vi "Stats Unbundle v0.2.vi"(8 "NAT Cluster in":T2, 9 "State":T4, 10 "Model":string, 11 "Auto Stats":T6) -> (0 "NAT Cluster out":T1, 1 "Cycle Time":dbl, 2 "Counters":cluster{"GoodCount":u32, "RejectCount":u32}, 3 "OEE Cluster":T3, 4 "Avg. Cycle Time":dbl, 5 "Total Times":T5, 7 "path":path)   [LabVIEW 2021]
doc: "v0.2:\n- Added state for saving and loading values"
uses:
  support/Controls/Auto Stats.ctl
  RT/Controls/Auto Times.ctl
  Controls/Logging FGV.ctl
  Controls/AVL Auto Time.ctl
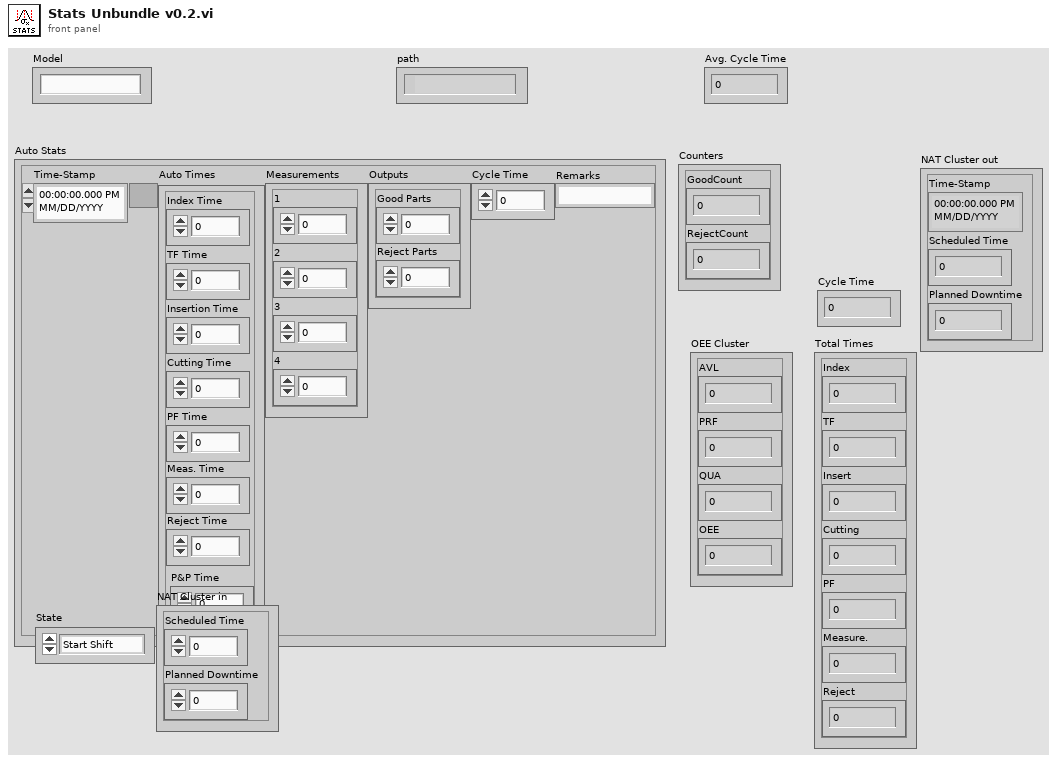
[diagram p1: front panel]
types:
  T1 = cluster{"Time-Stamp":timestamp, "Scheduled Time":dbl, "Planned Downtime":dbl}
  T2 = cluster{"Scheduled Time":dbl, "Planned Downtime":dbl}
  T3 = cluster{"AVL":dbl, "PRF":dbl, "QUA":dbl, "OEE":dbl}
  T4 = typedef "Logging FGV.ctl" = enum16{"Start Shift", "Reload Values", "Log Index", "Read Shift", "Close Shift", "Save Values"}
  T5 = cluster{"Index":dbl, "TF":dbl, "Insert":dbl, "Cutting":dbl, "PF":dbl, "Measure.":dbl, "Reject":dbl}
  T6 = typedef "Auto Stats.ctl" = cluster{"Time-Stamp":timestamp, "Auto Times":T7, "Measurements":cluster{"1":dbl, "2":dbl, "3":dbl, "4":dbl}, "Outputs":cluster{"Good Parts":u32, "Reject Parts":u32}, "Cycle Time":dbl, "Remarks":string}
  T7 = typedef "Auto Times.ctl" = cluster{"Index Time":u32, "TF Time":u32, "Insertion Time":u32, "Cutting Time":u32, "PF Time":u32, "Meas. Time":u32, "Reject Time":u32, "P&P Time":u32}
  T8 = typedef "AVL Auto Time.ctl" = enum16{"Start Session", "Exited Auto", "Resumed Auto", "Read Time", "Reload Values"}
  T9 = cluster{"[0]":dbl, "[1]":dbl, "[2]":dbl, "[3]":dbl, "[4]":dbl, "[5]":dbl, "[6]":dbl}
  T10 = cluster{"value":dbl, "value":dbl, "value":dbl, "value":dbl}
  T11 = cluster{"Time of Exit":timestamp, "value":dbl, "value":dbl}
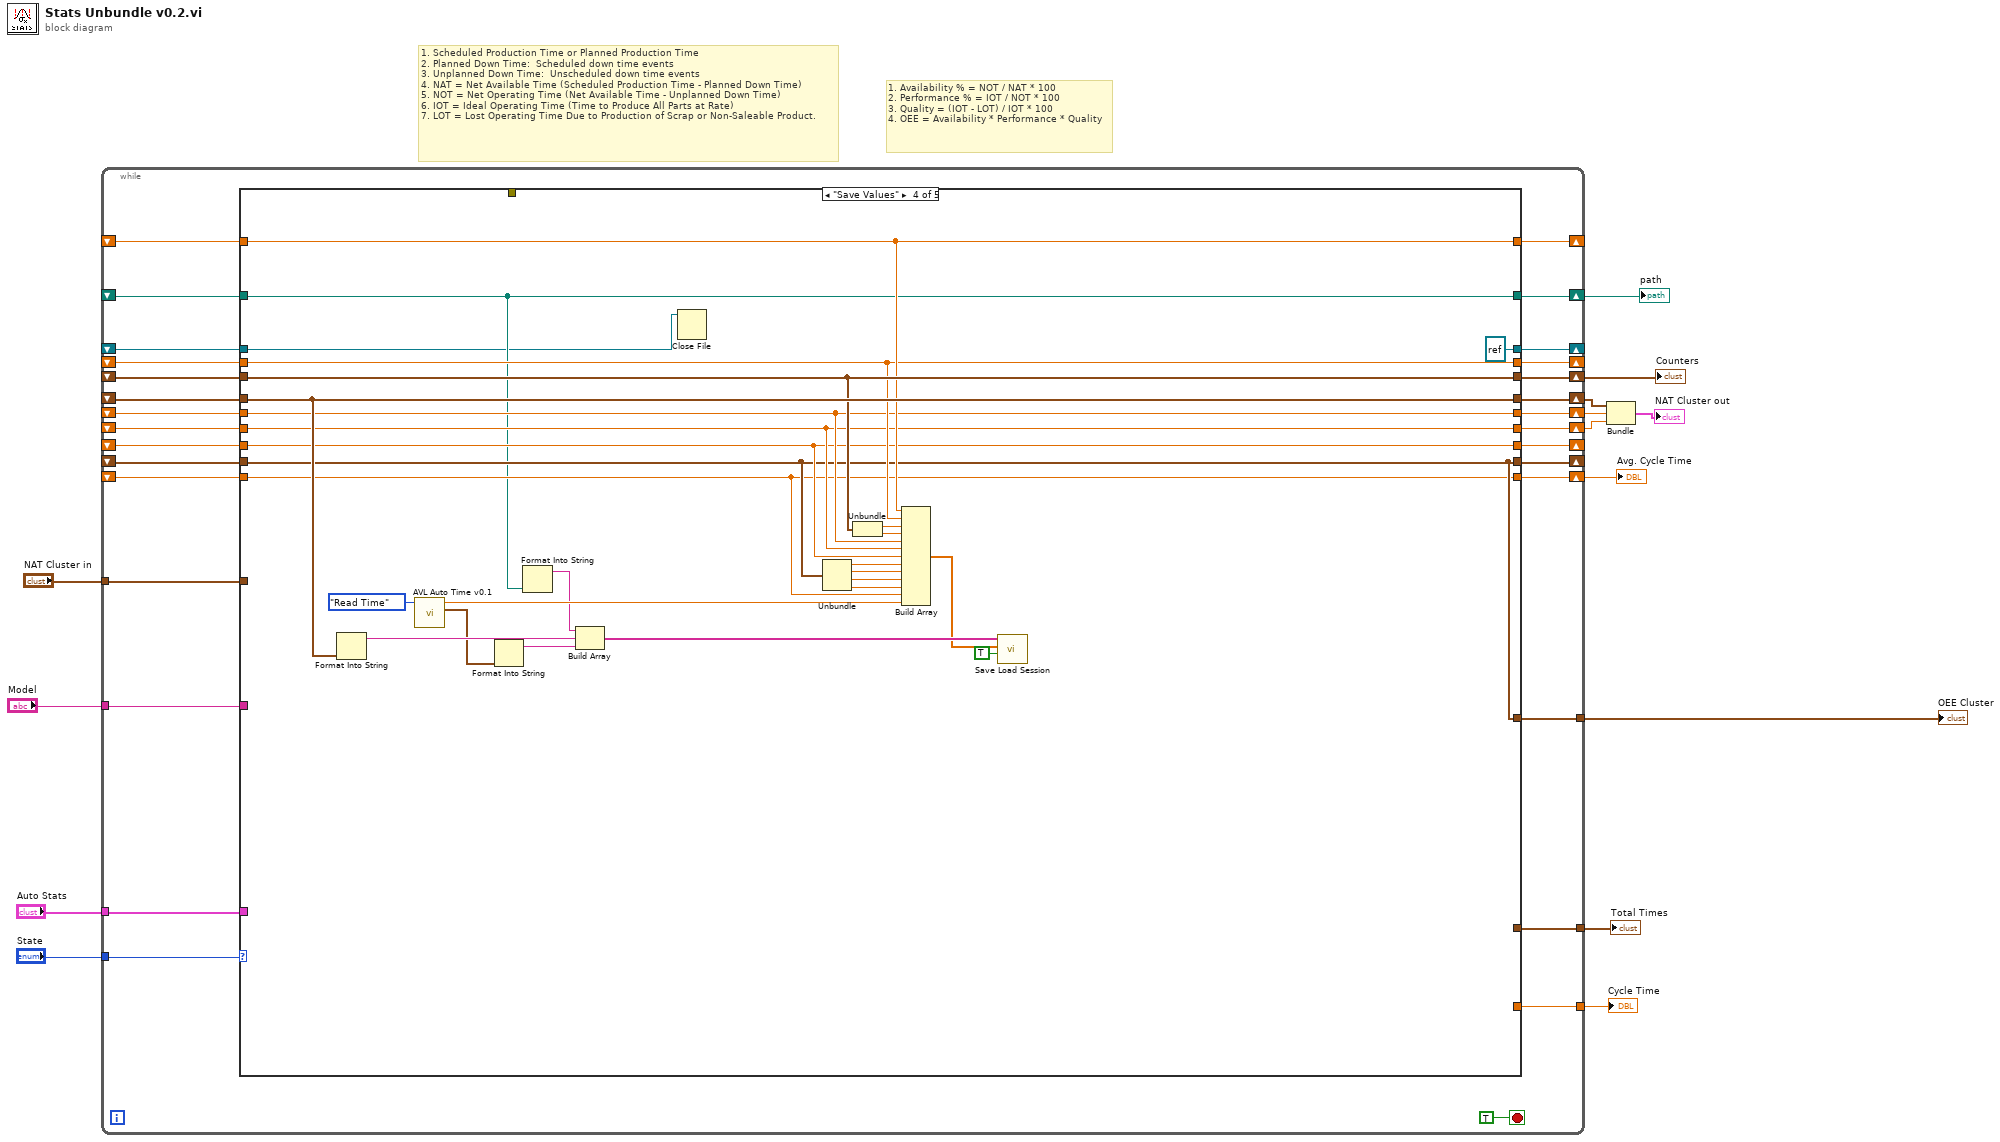
[diagram p0: block diagram]
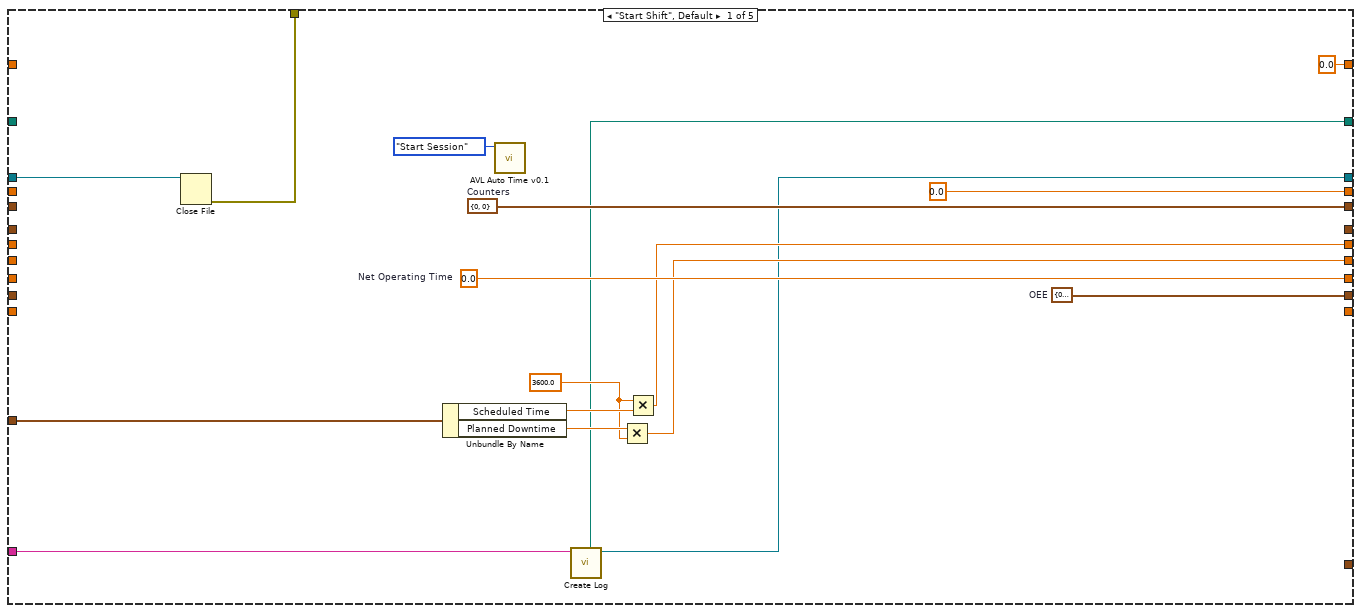
[diagram p2: hidden frame]
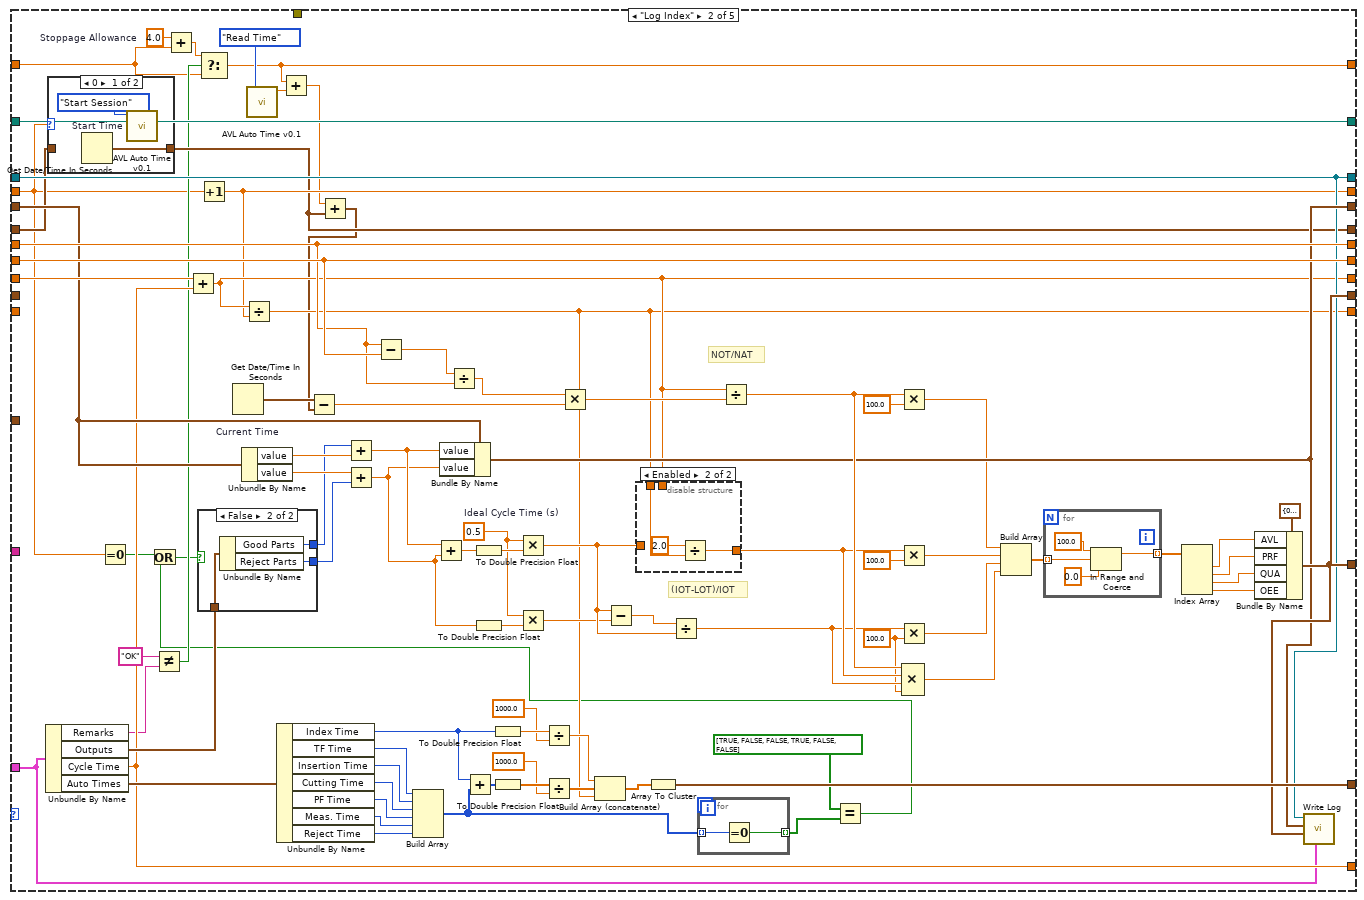
[diagram p3: hidden frame]
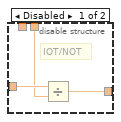
[diagram p4: hidden frame]
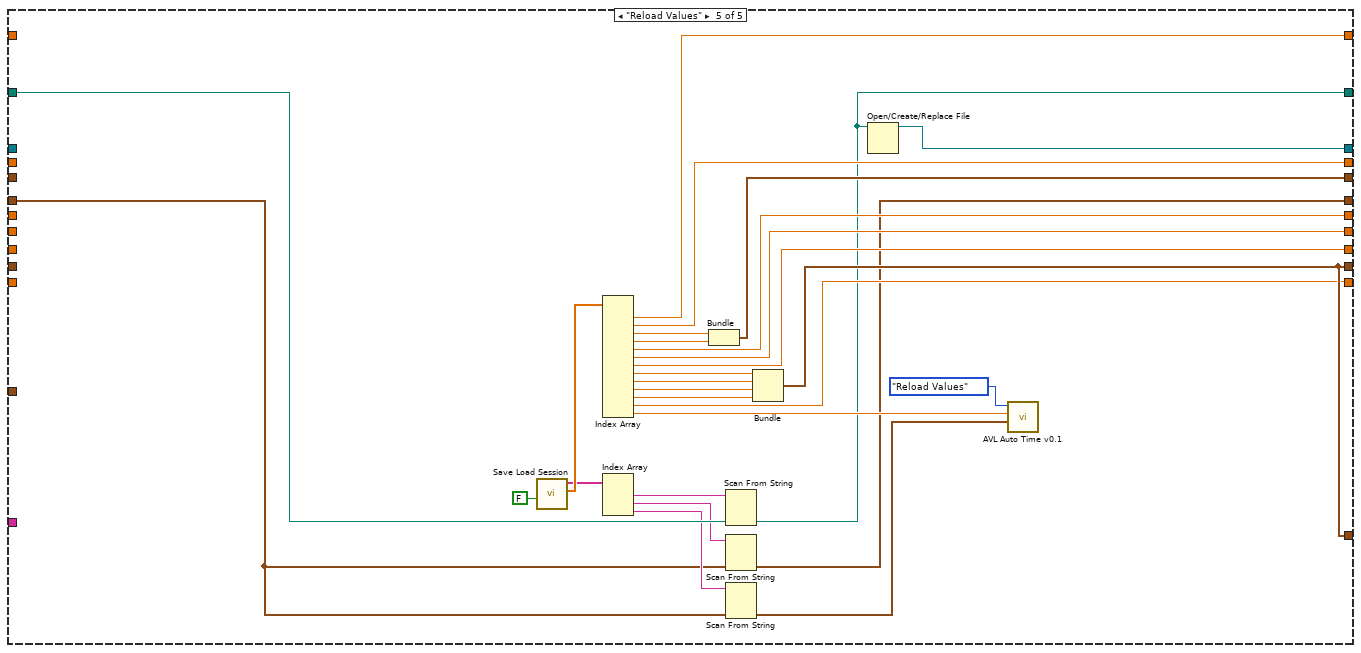
[diagram p8: hidden frame]
diagram:
  # "1.\tAvailability % = NOT / NAT * 100\n2.\tPerformance % = IOT / NOT * 100\n3.\tQuality = (IOT - LOT) / IOT * 100\n4.\tOEE = Availability * Performance * Quality"
  # "1.\tScheduled Production Time or Planned Production Time\n2.\tPlanned Down Time:  Scheduled down time events\n3.\tUnplanned Down Time:  Unscheduled down time events\n4.\tNAT = Net Available Time (Scheduled Production Time - Planned Down Time)\n5.\tNOT = Net Operating Time (Net Available Time - Unplanned Down Time)\n6.\tIOT = Ideal Operating Time (Time to Produce All Parts at Rate)\n7.\tLOT = Lost Operating Time Due to Production of Scrap or Non-Saleable Product."
  n1 = while {
    tunnel: "Auto Stats" -> [w44]
    tunnel: "State" -> [w43]
    shift-right: [w40] -> w8
    shift-left: _ -> [w37]
    shift-right: [w41] -> w9
    shift-left: _ -> [w38]
    shift-right: [w42] -> w6
    shift-left: _ -> [w39]
    shift-right: [w36] -> _
    shift-left: _ -> [w35]
    tunnel: [w34] -> w2
    shift-right: [w33] -> w13
    shift-left: _ -> [w32]
    tunnel: [w31] -> w12
    tunnel: [w29] -> w11
    shift-right: [w28] -> _
    shift-left: _ -> [w27]
    tunnel: "NAT Cluster in" -> [w26]
    shift-right: [w25] -> _
    shift-left: _ -> [w24]
    tunnel: "Model" -> [w23]
    shift-right: [w22] -> _
    shift-left: _ -> [w21]
    shift-right: [w20] -> w3
    shift-left: _ -> [w19]
    shift-right: [w18] -> w1
    shift-left: _ -> [w17]
    shift-right: [w16] -> _
    shift-left: _ -> [w15]
    stop <- TRUE stop-if-true
    n2 = case shown="\"Save Values\"" w43 {
      tunnel: w44 -> [_ w100 _ _ _]
      tunnel: [_ w79 w176 w202 w207] -> w42
      tunnel: [w54 w115 w173 w196 w222] -> w41
      tunnel: [w55 w130 w175 w195 w223] -> w40
      tunnel: w39 -> [_ w94 w176 w202 w204]
      tunnel: w38 -> [_ w115 w173 w196 _]
      tunnel: w37 -> [_ w130 w175 w195 _]
      tunnel: [w61 w96 w174 w194 w224] -> w36
      tunnel: w35 -> [_ w125 w174 w194 _]
      tunnel: [_ w99 w171 w193 w217] -> w34
      tunnel: [w60 w98 w172 w201 w225] -> w33
      tunnel: w32 -> [_ w105 w172 w201 _]
      tunnel: [_ w102 _ _ _] -> w31
      tunnel: [_ w101 _ _ _] -> w29
      tunnel: [w59 w99 w171 w193 w217] -> w28
      tunnel: w27 -> [_ _ w171 w193 _]
      tunnel: w26 -> [w56 _ _ _ _]
      tunnel: [w52 w97 w170 refnum<file> refnum ("refnum out") w209] -> w25
      tunnel: w24 -> [w51 w97 w170 w178 _]
      tunnel: [w50 _ _ _ _] -> _
      tunnel: w23 -> [w49 _ _ _ _]
      tunnel: [0.0 w95 w169 w199 w228] -> w22
      tunnel: w21 -> [_ w65 w169 w199 _]
      tunnel: [_ w80 w168 w188 w216] -> w20
      tunnel: w19 -> [_ _ w168 w188 _]
      tunnel: [w47 w83 w167 w186 w210] -> w18
      tunnel: w17 -> [_ w83 w167 w186 w211]
      tunnel: [0.0 w70 w166 w200 w229] -> w16
      tunnel: w15 -> [_ w72 w166 w200 _]
      frame "Start Shift", Default {
        w53 = 3600.0 ("y")
        w59 = T3 {"AVL"=0.0, "PRF"=0.0, "QUA"=0.0, "OEE"=0.0}  # OEE
        w60 = cluster{"GoodCount":u32, "RejectCount":u32} {"GoodCount"=0, "RejectCount"=0}  # Counters
        w61 = 0.0  # Net Operating Time
        n3 = Close File(refnum=w51) -> (error out=w50:errorcluster)  [unwired: 1 in, 1 out]
        n4 = Unbundle By Name(w56) -> ("Scheduled Time"=w58:dbl, "Planned Downtime"=w57:dbl)
        n5 = call "AVL Auto Time v0.1.vi"("State"=AVL_Auto_Time."Start Session") -> ()  [unwired: 9 in, 2 out]
        n6 = call "Create Log.vi"("Model"=w49) -> ("refnum out"=w52:refnum<file>, "path"=w47:path)  [unwired: 9 in]
        n7 = Multiply(x=w57, y=w53) -> (x*y=w55:dbl)
        n8 = Multiply(x=w53, y=w58) -> (x*y=w54:dbl)
      }
      frame "Log Index" {
        w75 = 4.0  # Stoppage Allowance
        w111 = 100.0 ("y")
        w116 = 0.5  # Ideal Cycle Time (s)
        # "NOT/NAT"
        # "(IOT-LOT)/IOT"
        n9 = Unbundle By Name(w100) -> ("Remarks"=w77:string, "Outputs"=w124:cluster{"Good Parts":u32, "Reject Parts":u32}, "Cycle Time"=w102:dbl, "Auto Times"=w147:T7)
        n10 = case shown="0" w65 {
          tunnel: w94 -> [_ w165]
          tunnel: [w164 w165] -> w79
          frame 0 {
            n11 = Get Date/Time In Seconds "Start Time"() -> (seconds since 1Jan1904=w164:timestamp)
            n12 = call "AVL Auto Time v0.1.vi"("State"=AVL_Auto_Time."Start Session") -> ()  [unwired: 9 in, 2 out]
          }
          frame Default {
          }
        }
        n13 = Equal To 0?(x=w65) -> (x = 0?=w64:bool)
        n14 = Not Equal?(x="OK", y=w77) -> (x != y?=w74:bool)
        n15 = Add(x=w75, y=w72) -> (x+y=w73:dbl)
        n16 = Add(x=w125, y=w102) -> (x+y=w96:dbl)
        n17 = Select(t=w73, s=w74, f=w72) -> (s? t:f=w70:dbl)
        n18 = Increment(x=w65) -> (x+1=w95:dbl)
        n19 = Get Date/Time In Seconds "Current Time"() -> (seconds since 1Jan1904=w131:timestamp)
        n20 = Unbundle By Name(w105) -> ("value"=w109:dbl, "value"=w108:dbl)
        n21 = Divide(x=w96, y=w95) -> (x/y=w80:dbl)
        n22 = call "AVL Auto Time v0.1.vi"("State"=AVL_Auto_Time."Read Time") -> ("Non-Auto Time"=w71:dbl)  [unwired: 9 in, 1 out]
        n23 = Unbundle By Name(w147) -> ("Index Time"=w133:u32, "TF Time"=w141:u32, "Insertion Time"=w142:u32, "Cutting Time"=w143:u32, "PF Time"=w144:u32, "Meas. Time"=w145:u32, "Reject Time"=w146:u32)
        n24 = Add(x=w70, y=w71) -> (x+y=w69:dbl)
        n25 = Add(x=w69, y=w79) -> (x+y=w78:timestamp)
        n26 = Subtract(x=w131, y=w78) -> (x-y=w129:dbl)
        n27 = Subtract(x=w115, y=w130) -> (x-y=w128:dbl)
        n28 = Build Array(w141, w142, w143, w144, w145, w146) -> (w68:u32[])
        n29 = Divide(x=w128, y=w115) -> (x/y=w82:dbl)
        n30 = Add(x=w133, y=w68) -> (x+y=w138:u32[])
        n31 = To Double Precision Float(number=w133) -> (double precision float=w135:dbl)
        n32 = To Double Precision Float(number=w138) -> (double precision float=w140:dbl[])
        n33 = Divide(x=w135, y=1000.0) -> (x/y=w132:dbl)
        n34 = Divide(x=w140, y=1000.0) -> (x/y=w137:dbl[])
        n35 = Multiply(x=w82, y=w129) -> (x*y=w126:dbl)
        n36 = Build Array (concatenate)(w132, w137, w80) -> (w136:dbl[])
        n37 = Array To Cluster(array=w136) -> (cluster=w101:T9)
        n38 = for {
          tunnel: w68 -> [w149] mode=indexing
          tunnel: [w148] -> w67 mode=indexing
          n39 = Equal To 0?(x=w149) -> (x = 0?=w148:bool)
        }
        n40 = Divide(x=w96, y=w126) -> (x/y=w114:dbl)
        n41 = Equal?(x=bool[] [TRUE, FALSE, FALSE, TRUE, FALSE, FALSE], y=w67) -> (x = y?=w63:bool)
        n42 = Or(x=w64, y=w63) -> (x .or. y?=w62:bool)
        n43 = case shown="False" w62 {
          tunnel: w124 -> [_ w160]
          tunnel: [_ w162] -> w107
          tunnel: [_ w161] -> w106
          frame True {
          }
          frame False {
            n44 = Unbundle By Name(w160) -> ("Good Parts"=w162:u32, "Reject Parts"=w161:u32)
          }
        }
        n45 = Add(x=w107, y=w109) -> (x+y=w104:dbl)
        n46 = Add(x=w108, y=w106) -> (x+y=w103:dbl)
        n47 = Add(x=w104, y=w103) -> (x+y=w123:dbl)
        n48 = Bundle By Name(cluster=w105, "value"=w104, "value"=w103) -> (w98:cluster{"value":dbl, "value":dbl})
        n49 = To Double Precision Float(number=w123) -> (double precision float=w122:dbl)
        n50 = To Double Precision Float(number=w103) -> (double precision float=w120:dbl)
        n51 = Multiply(x=w116, y=w122) -> (x*y=w118:dbl)
        n52 = Multiply(x=w116, y=w120) -> (x*y=w117:dbl)
        n53 = Subtract(x=w118, y=w117) -> (x-y=w119:dbl)
        n54 = disable-structure shown="Enabled" {
          disable-tunnel: w118 -> [w152 _]
          disable-tunnel: [w151 w153] -> w113
          disable-tunnel: w96 -> [w150 _]
          disable-tunnel: w80 -> [_ w155]
          frame Disabled {
            # "IOT/NOT"
            n55 = Divide(x=w152, y=w150) -> (x/y=w151:dbl)
          }
          frame Enabled {
            n56 = Divide(x=2.0 ("y"), y=w155) -> (x/y=w153:dbl)
          }
        }
        n57 = Divide(x=w119, y=w118) -> (x/y=w112:dbl)
        n58 = Multiply(x=w114, y=100.0) -> (x*y=w93:dbl)
        n59 = Multiply(x=w113, y=100.0) -> (x*y=w92:dbl)
        n60 = Multiply(x=w112, y=w111) -> (x*y=w91:dbl)
        n61 = Compound Arithmetic op=MULTIPLY(w114, w113, w112, w111) -> (w90:dbl)
        n62 = Build Array(w93, w92, w91, w90) -> (w89:dbl[])
        n63 = for {
          tunnel: w89 -> [w157] mode=indexing
          tunnel: [w156] -> w88 mode=indexing
          n64 = In Range and Coerce(upper limit=100.0, x=w157, lower limit=0.0) -> (coerced(x)=w156:dbl)  [unwired: 1 out]
        }
        n65 = Index Array(array=w88) -> (element #1=w87:dbl, element #2=w86:dbl, element #3=w85:dbl, element #4=w84:dbl)  [unwired: 4 in]
        n66 = Bundle By Name(cluster=T3 {"AVL"=0.0, "PRF"=0.0, "QUA"=0.0, "OEE"=0.0} ("OEE 2"), "AVL"=w87, "PRF"=w86, "QUA"=w85, "OEE"=w84) -> (w99:T3)
        n67 = call "Write Log.vi"("Auto Stats"=w100, "OEE in"=w99, "output cluster"=w98, "refnum out"=w97) -> ()  [unwired: 8 in]
      }
      frame "Read Shift" {
      }
      frame "Save Values" {
        n68 = Format Into String(w202) -> (resulting string=w184:string)  [unwired: 3 in, 1 out]
        n69 = call "AVL Auto Time v0.1.vi"("State"=AVL_Auto_Time."Read Time") -> ("Time of Exit"=w183:timestamp, "Non-Auto Time"=w187:dbl)  [unwired: 9 in]
        n70 = Format Into String(w183) -> (resulting string=w182:string)  [unwired: 3 in, 1 out]
        n71 = Format Into String(w186) -> (resulting string=w185:string)  [unwired: 3 in, 1 out]
        n72 = Build Array(w185, w184, w182) -> (w181:string[])
        n73 = Close File(refnum=w178) -> ()  [unwired: 1 in, 2 out]
        n74 = Unbundle(w193) -> ("value"=w192:dbl, "value"=w191:dbl, "value"=w190:dbl, "value"=w189:dbl)
        n75 = Unbundle(w201) -> ("value"=w198:dbl, "value"=w197:dbl)
        n76 = Build Array(w200, w199, w198, w197, w196, w195, w194, w192, w191, w190, w189, w188, w187) -> (w180:dbl[])
        n77 = call "Save Load Session.vi"("Write"=TRUE, "Numeric Array In"=w180, "Str Array in"=w181) -> ()  [unwired: 7 in, 2 out]
      }
      frame "Reload Values" {
        n78 = call "Save Load Session.vi"("Write"=FALSE) -> ("Numeric Array Out"=w230:dbl[], "Str Array out"=w213:string[])  [unwired: 9 in]
        n79 = Index Array(array=w230) -> (element #1=w229:dbl, element #2=w228:dbl, element #3=w227:dbl, element #4=w226:dbl, element #5=w222:dbl, element #6=w223:dbl, element #7=w224:dbl, element #8=w221:dbl, element #9=w220:dbl, element #10=w219:dbl, element #11=w218:dbl, element #12=w216:dbl, element #13=w214:dbl)  [unwired: 13 in]
        n80 = Index Array(array=w213) -> (element #1=w212:string, element #2=w208:string, element #3=w206:string)  [unwired: 3 in]
        n81 = Bundle("value"=w227, "value"=w226) -> (w225:cluster{"value":dbl, "value":dbl})  [unwired: 1 in]
        n82 = Scan From String(input string=w212, default 1=w211) -> (output 1=w210:path)  [unwired: 3 in, 3 out]
        n83 = Scan From String(input string=w208, default 1=w204) -> (output 1=w207:timestamp)  [unwired: 3 in, 3 out]
        n84 = Scan From String(input string=w206, default 1=w204) -> (output 1=w205:timestamp)  [unwired: 3 in, 3 out]
        n85 = Bundle("value"=w221, "value"=w220, "value"=w219, "value"=w218) -> (w217:T10)  [unwired: 1 in]
        n86 = Open/Create/Replace File(file path (use dialog)=w210) -> (refnum out=w209:refnum<file>)  [unwired: 5 in, 2 out]
        n87 = call "AVL Auto Time v0.1.vi"("Time of Exit in"=w205, "Non-Auto Time in"=w214, "State"=AVL_Auto_Time."Reload Values") -> ()  [unwired: 7 in, 2 out]
      }
    }
  }
  "OEE Cluster" <- w2
  "Counters" <- w13
  "Cycle Time" <- w12
  "Total Times" <- w11
  "Avg. Cycle Time" <- w3
  "path" <- w1
  n88 = Bundle("Time of Exit"=w6, "value"=w9, "value"=w8) -> (→"NAT Cluster out":T11)  [unwired: 1 in]
